vi "CoSim.vi"() -> ()   [LabVIEW 2015]
uses:
  SVPWM/Parameters.ctl
  <vilib>/Simulation/Scripting/Companion Diagram/SimConfigNode/SimParams.ctl
  <vilib>/Simulation/Scripting/Companion Diagram/SimConfigNode/_simSolvers.ctl
  <vilib>/Simulation/Implementation/Shared/SIMSCR Execution Mode.ctl
  <vilib>/Simulation/Param Hierarchy/Typedefs/SIMPH Param Control Actions.ctl
  <vilib>/Simulation/Scripting/Editor Utilities/SIM subVI tag data.ctl
  <vilib>/Simulation/Scripting/Editor Utilities/SIM subVI execution type.ctl
  <vilib>/Utility/error.llb/Clear Errors.vi
  <vilib>/rvi/Emulation/niFpgaSctlEmulationGetInTimedLoop.vi
  <vilib>/Simulation/Implementation/Shared/NILVSim_ParamChanged.vi
  <vilib>/Simulation/Implementation/Shared/NILVSIM_BeginStep.vi
  <vilib>/Simulation/DataSources/Implementation/NILVSim Sine Wave.llb/SIM Sine Wave (scalar).vi
  <vilib>/Simulation/Utility/Implementation/SIM Halt.vi
  <vilib>/Simulation/Utility/Implementation/SIM Time.vi
  <vilib>/Simulation/Implementation/Shared/SIM Fire Discrete SubVI.vi
  <vilib>/Simulation/Implementation/Shared/NILVSim_Manager.vi
  <vilib>/Simulation/Implementation/Shared/NILVSim_FinalizeModel.vi
  <vilib>/Simulation/Implementation/Shared/SIM Fire Discrete SubVI (Core).vi
  <vilib>/rvi/DataTransferAndStorage/Container/Common/niFpgaContainerGetUniqueNameForEmu.vi
  <vilib>/rvi/DataTransferAndStorage/Container/Common/niFpgaContainerSetEmuInfo.vi
  <vilib>/rvi/eio/common/nirviEmuReportErrorAndStop.vi
  <vilib>/rvi/DataTransferAndStorage/Container/Common/niFpgaContainerExecOnDevCompGetState.vi
  <vilib>/rvi/Emulation/niFpgaEmulationIsFPGAContextNoSignature.vi
  <vilib>/rvi/Memory/Memory_Emulation/niFpgaMemoryEmulationCacheClearOnFirstRun.vi
  <vilib>/rvi/Memory/Memory_Emulation/nirvimemoryEmulationManagerCache_MakeExclusive.vi
  <vilib>/rvi/Memory/Memory_Emulation/niFpgaMemoryEmulationValidateCache.vi
  <vilib>/rvi/Memory/Memory_Emulation/nirvimemoryEmulationManagerCache_InsertValue.vi
  <vilib>/rvi/Memory/Memory_Emulation/nirvimemoryEmulationManagerCache_ReleaseExclusive.vi
  <vilib>/rvi/Memory/Memory_Emulation/nirvimemoryEmulationManagerCache_GetValue.vi
  <vilib>/rvi/Memory/Memory_Emulation/nirvimemoryEmulationManagerCache_SetValue.vi
  <vilib>/rvi/Emulation/niFpgaProcessEmulError.vi
  <vilib>/Simulation/Implementation/Shared/SIM Unbundle Sim Info.vi
  <vilib>/Simulation/Implementation/Shared/NILVSim_Initialize.vi
  <vilib>/Simulation/Utility/Implementation/NILVSim Get Time and IsAcceptedStep.vi
  Transforms/dev/_IPBuilder/ABCtoAlphaBeta_src.vi
  Transforms/dev/_IPBuilder/AlphaBetaAndDQ_variants/ABCtoAlphaBeta_3PhaseUnitaryMagnitude_src.vi
  multirateCosimSVPWM.vi
  <vilib>/Simulation/Implementation/Shared/SIMSH Read Queue.vi
  <vilib>/Simulation/Implementation/Shared/NILVSim_GetModelError.vi
  <vilib>/Simulation/Implementation/Shared/SIM Bundle Sim Info.vi
  <vilib>/Simulation/Scripting/Companion Diagram/SimConfigNode/SimDog.xnode
  <vilib>/rvi/LocalResourceManager/LocalResourceManager.xnode
  <vilib>/rvi/DataTransferAndStorage/Container/XNode/niFpgaContainer.xnode
  <vilib>/rvi/DataTransferAndStorage/Register/Emulation/niFpgaRegisterEmulationRefIn.vi
  <vilib>/Simulation/Implementation/XNodeFramework/SimXNode/SimX.xnode
  <vilib>/Simulation/EMI/Plugins/Multisim Design/MultisimEMICtrl.dll
  SVPWMInterface/SVPWMInterface.lvlib
  <vilib>/Simulation/Implementation/Shared/NI_SIM_Implementation.lvlib
  SVPWM/SVPWM.lvlib
panel:
  out "simulation time":dbl
  in  "Halt?":bool
  in  "frequency":dbl=0.5
  in  "amplitude":dbl=1.0
  out "Signals":dbl[][](graph)
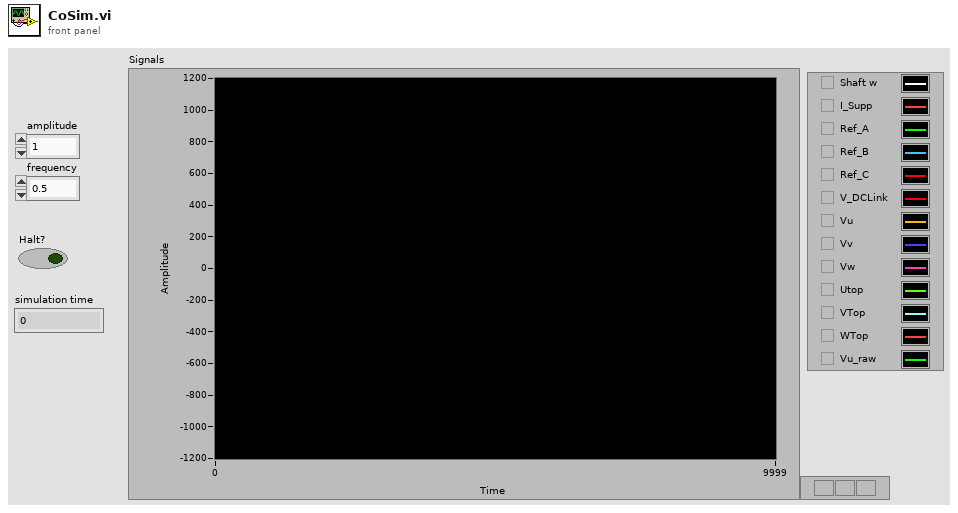
[diagram p1: front panel]
types:
  T1 = typedef "SVPWM.lvlib/Parameters.ctl" = cluster{"Deadtime":refnum<k21>, "Period":refnum<k21>}
  T2 = typedef "SVPWMInterface.lvlib/Configuration.ctl" = cluster{"Deadtime":u8, "Period":u32}
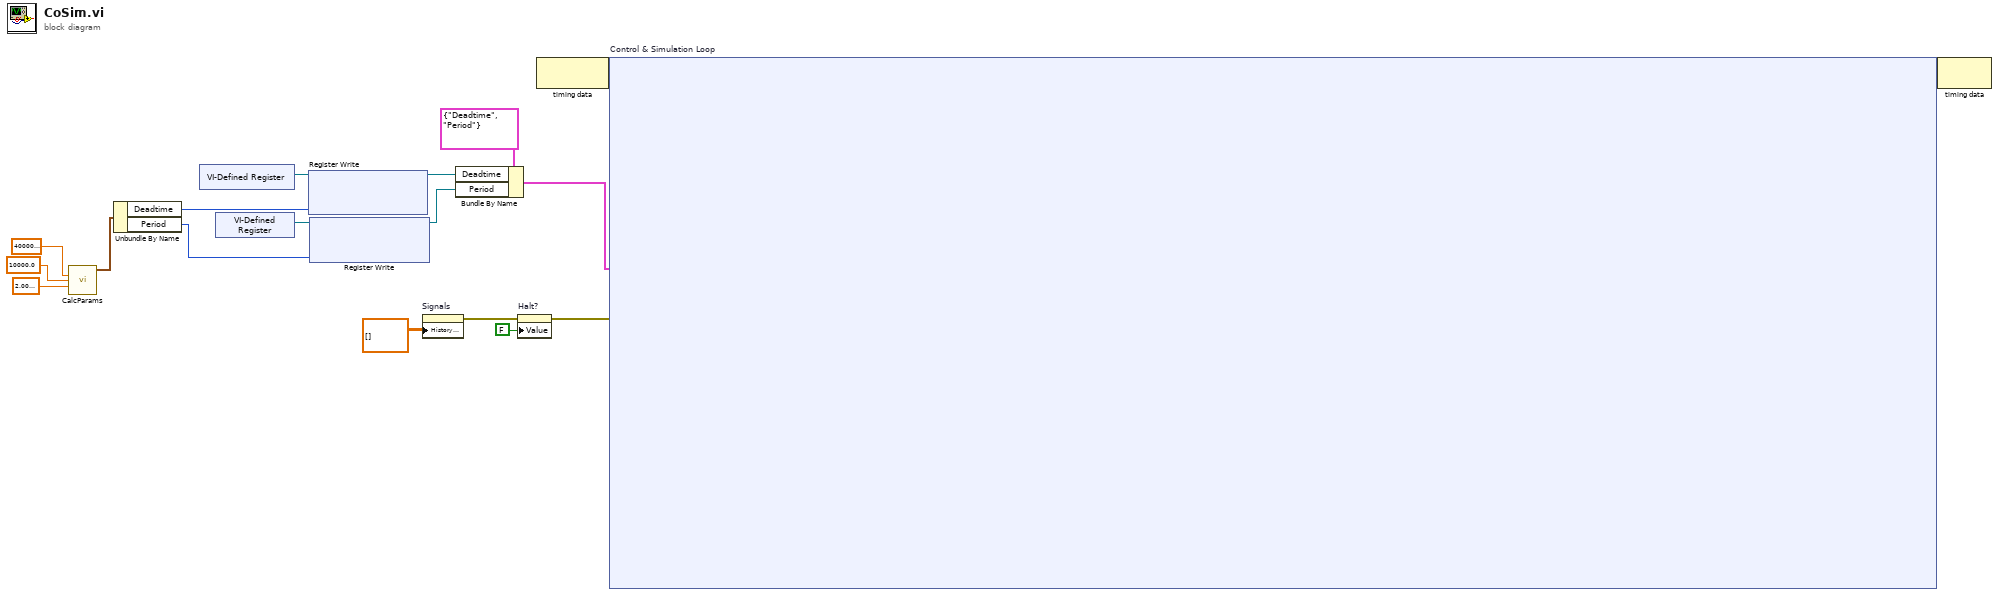
[diagram p0: block diagram]
diagram:
  n1 = call "CalcParams.vi"("ClkRate"=sgl 40000000.0, "fc"=sgl 10000.0, "deadtime"=sgl 2e-07) -> ("Configuration"=w4:T2)  [unwired: 12 in]
  n2 = Unbundle By Name(w4) -> ("Deadtime"=w3:u8, "Period"=w2:u32)
  n3 = xnode "VI-Defined Register"() -> ("Register Out"=w8:refnum<k21>)
  n4 = xnode "VI-Defined Register"() -> ("Register Out"=w6:refnum<k21>)
  n5 = xnode ("Register Write")("Data"=w3, "Register In"=w8) -> ("Register Out"=w7:refnum<k21>)
  n6 = xnode ("Register Write")("Data"=w2, "Register In"=w6) -> ("Register Out"=w5:refnum<k21>)
  n7 = property on="Signals" class="WFChart (strict)"("History Data"=dbl[][] []) -> (error out=w12:errorcluster)  [unwired: 2 in, 1 out]
  n8 = Bundle By Name(cluster=T1 {"Deadtime"="Deadtime", "Period"="Period"} ("SVPWM_SGL"), "Deadtime"=w7, "Period"=w5) -> (w1:T1)
  n9 = property on="Halt?" class="Bool (strict)"(error in=w12, "Value"=FALSE ("Halt?")) -> (error out=w10:errorcluster)  [unwired: 1 in, 1 out]
  n10 = node-c288() -> (w18:variant)  [unwired: 1 in]
  n11 = node-c254 "Control & Simulation Loop"(w18, w1, w10) -> (w17:variant)
  n12 = node-c288(w17) -> ()  [unwired: 1 out]
